vi "Load Connection File.vi"(8 "error in (no error)":errorcluster, 11 "Path to Connection File":path) -> (0 "error out":errorcluster, 3 "Connection Info":T1)   [LabVIEW 2018, in "ClientMessaging.lvlib"]
uses:
  ClientMessaging.lvlib
  Connection.ctl
  <vilib>/Utility/sysdir.llb/System Directory Type.ctl
  <vilib>/JDP Science/JSONtext/JSONtext.lvlib
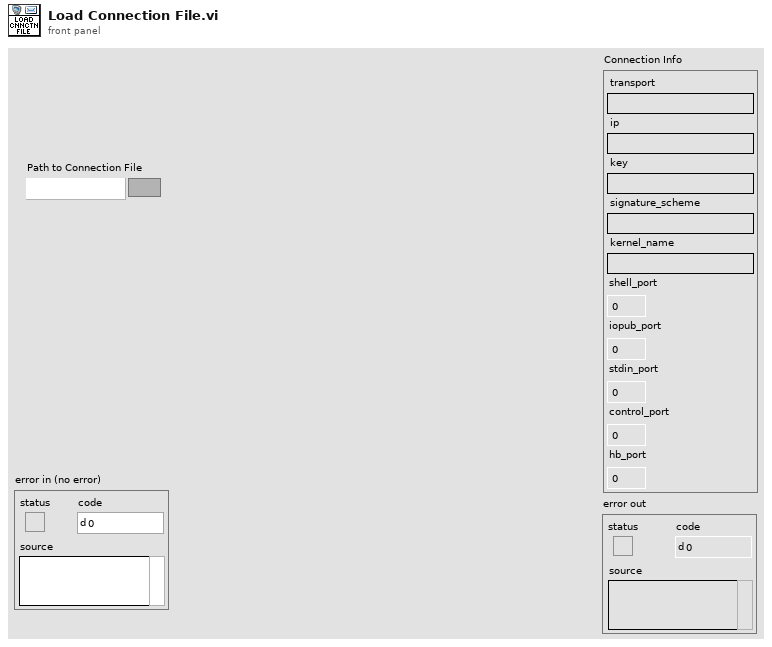
[diagram p1: front panel]
types:
  T1 = typedef "ClientMessaging.lvlib/Connection.ctl" = cluster{"transport":string, "ip":string, "key":string, "signature_scheme":string, "kernel_name":string, "shell_port":u16, "iopub_port":u16, "stdin_port":u16, "control_port":u16, "hb_port":u16}
  T2 = typedef "System Directory Type.ctl" = i32
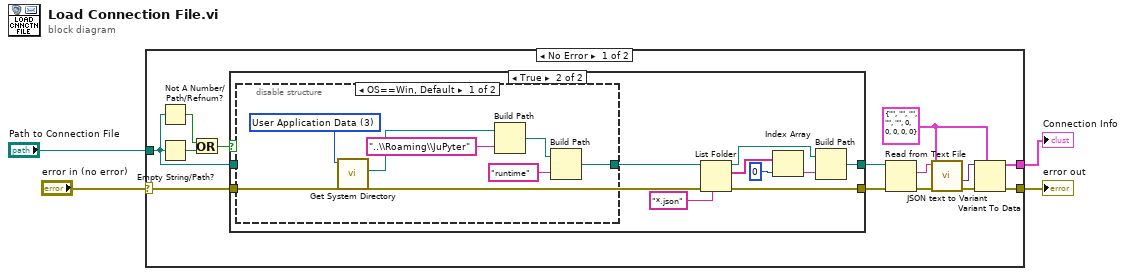
[diagram p0: block diagram]
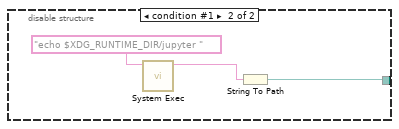
[diagram p3: hidden frame]
diagram:
  n1 = case shown="No Error" "error in (no error)" {
    selector: "error in (no error)" -> [w11 w39]
    tunnel: [w10 w39] -> w3
    tunnel: "Path to Connection File" -> [w13 _]
    tunnel: [w12 _] -> w1
    frame No Error {
      w8 = T1 {"transport"="", "ip"="", "key"="", "signature_scheme"="", "kernel_name"="", "shell_port"=0, "iopub_port"=0, "stdin_port"=0, "control_port"=0, "hb_port"=0} ("Connection Info")
      n2 = Not A Number/Path/Refnum?(number/path/refnum=w13) -> (NaN/Path/Refnum?=w18:bool)
      n3 = Empty String/Path?(string/path=w13) -> (empty?=w16:bool)
      n4 = Or(x=w18, y=w16) -> (x .or. y?=w17:bool)
      n5 = case shown="True" w17 {
        tunnel: w11 -> [w19 w23]
        tunnel: [w19 w22] -> w15
        tunnel: [w20 w21] -> w14
        tunnel: w13 -> [w20 _]
        frame False {
        }
        frame True {
          n6 = disable-structure shown="OS==Win, Default" {
            disable-tunnel: [w35 w36] -> w29
            frame condition #0 (active) {
              w31 = T2 3 items=["User Home"=0, "User Desktop"=1, "User Documents"=2, "User Application Data"=3, "User Preferences"=4, "User Temporary"=5, "Public Documents"=6, "Public Application Data"=7, "Public Preferences"=8, "Public Cache"=13, "System Core Libraries"=9, "System Installed Libraries"=10, "Application Files"=11, "Boot Volume Root"=12] ("system directory type")
              n7 = call <vilib>:"Get System Directory.vi"("system directory type"=w31) -> ("system directory"=w30:path)  [unwired: 10 in]
              n8 = Build Path(base path=w30, name or relative path="..\\Roaming\\JuPyter") -> (appended path=w33:path)
              n9 = Build Path(base path=w33, name or relative path="runtime") -> (appended path=w35:path)
            }
            frame condition #1 {
              n10 = call <vilib>:"System Exec.vi"("command line"="echo $XDG_RUNTIME_DIR/jupyter ") -> ("standard output"=w37:string)  [unwired: 7 in, 3 out]
              n11 = String To Path(string=w37) -> (path=w36:path)
            }
          }
          n12 = List Folder(path=w29, pattern="*.json", error in=w23) -> (path out=w24:path, filenames=w27:string[], error out=w22:errorcluster)  [unwired: 1 in, 1 out]
          n13 = Index Array(array=w27, index=0) -> (element=w25:string)
          n14 = Build Path(base path=w24, name or relative path=w25) -> (appended path=w21:path)
        }
      }
      n15 = Read from Text File(file (use dialog)=w14, error in=w15) -> (text=w9:string, error out=w6:errorcluster)  [unwired: 2 in, 2 out]
      n16 = call <vilib>:"JSON text to Variant.vi"("error in (no error)"=w6, "Data Type"=w8, "JSON"=w9) -> ("error out"=w5:errorcluster, "Variant out"=w7:variant)  [unwired: 7 in]
      n17 = Variant To Data(error in=w5, type=w8, Variant=w7) -> (data=w12:T1, error out=w10:errorcluster)
    }
    frame Error {
    }
  }
  "error out" <- w3
  "Connection Info" <- w1
